vi "I2C_WriteSlaveDeviceAddress_2.vi"(5 "PostAddressDelay(Ticks)":u32, 7 "HalfCycle(Ticks)":u32, 8 "error in":errorcluster, 9 "R/W_Bit":bool, 10 "10-Bit Address":bool, 11 "AddressBits":u8[](array[numeric])=[0, 0] caption="AddressBytes" format="%.0x") -> (0 "error out":errorcluster, 2 "Status":i16)   [LabVIEW 2019]
doc: "Writes the Slave Device Address Byte (w/the R/W Bit set) out the I2C Bus\n\n<b>Inputs:</b>\n---------------------\n<b>AddressBytes</b> the address of the slave device that the master wants to communicate with.\n\n<b>10-Bit Address</b> boolean control for enabling 10-Bit sddressing scheme (True = Use 10-Bit address)\n\n<b>R/W_Bit</b> boolean control for setting the read or write bit (True=Read, =1)\n\n<b>HalfCycle(Ticks)</b> this the number of FPGA clock cycles in half og the clock period. Therefore twice this number yields the clock period, in ticks.\n\n<b>PostAddressDelay(Ticks)</b> the delay in FPGA clock cycles before writing bytes on SDA.\n\n<b>Outputs:</b>\n---------------------\n<b>Status</b> returns a numeric value representing the status of the I2C bus / slave device.\n0 = slave responded\n5002 = slave did not respond\n\nSee block diagram for more details on the implementation details.\n\nAuthor:\nPeter Fuller\nSenior Engineer\nPLF Consulting, LLC\n\nemail: peter@plfconsulting.com\nphone: 617.699.2201"
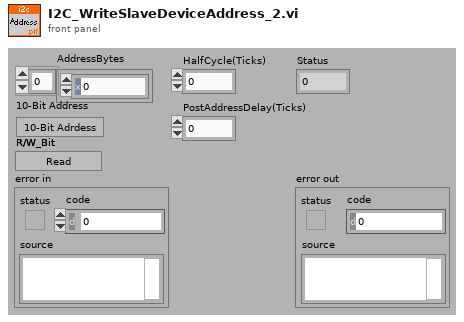
[diagram p1: front panel]
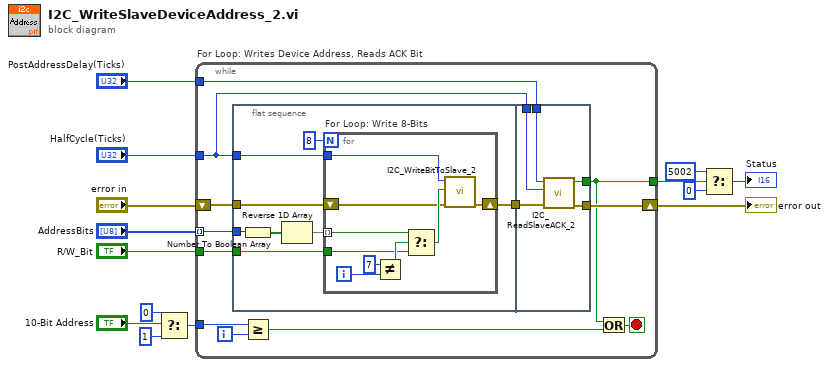
[diagram p0: block diagram]
diagram:
  n1 = Select(t=0, s="10-Bit Address", f=1) -> (s? t:f=w9:i32)
  n2 = while "For Loop: Writes Device Address, Reads ACK Bit" {
    tunnel: "HalfCycle(Ticks)" -> [w18]
    shift-right: [w16] -> w13
    shift-left: "error in" -> [w26]
    tunnel: "AddressBits" -> [w25] mode=indexing
    tunnel: [w15] -> w2
    tunnel: w9 -> [w20]
    tunnel: "R/W_Bit" -> [w19]
    tunnel: "PostAddressDelay(Ticks)" -> [w17]
    i -> [w24]
    stop <- w23 stop-if-true
    n3 = flat-sequence {
      tunnel: w18 -> [w28]
      tunnel: w26 -> [w30]
      tunnel: w25 -> [w33]
      tunnel: [w29] -> w21
      tunnel: w19 -> [w27]
      tunnel: w21 -> [w46]
      tunnel: w18 -> [w48]
      tunnel: w17 -> [w47]
      tunnel: [w45] -> w16
      tunnel: [w44] -> w15
      frame #0 {
        n4 = Number To Boolean Array(number=w33) -> (Boolean array=w32:bool[])
        n5 = Reverse 1D Array(array=w32) -> (reversed array=w31:bool[])
        n6 = for "For Loop: Write 8-Bits" {
          N: 8 -> [_]
          tunnel: w31 -> [w40] mode=indexing
          shift-right: [w35] -> w29
          shift-left: w30 -> [w36]
          tunnel: w28 -> [w43]
          tunnel: w27 -> [w37]
          i -> [w42]
          n7 = Not Equal?(x=7, y=w42) -> (x != y?=w38:bool)
          n8 = Select(t=w40, s=w38, f=w37) -> (s? t:f=w39:bool)
          n9 = call "I2C_WriteBitToSlave_2.vi"("error in"=w36, "Bit_Value"=w39, "HalfCycle(Ticks)"=w43) -> ("error out"=w35:errorcluster)  [unwired: 8 in]
        }
      }
      frame #1 {
        n10 = call "I2C_ReadSlaveACK_2.vi"("error in"=w46, "HalfCycle(Ticks)"=w48, "InterByteTransmitDelay(Ticks)"=w47) -> ("error out"=w45:errorcluster, "SDA"=w44:bool)  [unwired: 7 in]
      }
    }
    n11 = Greater Or Equal?(x=w20, y=w24) -> (x >= y?=w22:bool)
    n12 = Or(x=w15, y=w22) -> (x .or. y?=w23:bool)
  }
  "error out" <- w13
  n13 = Select(t=i16 5002, s=w2, f=i16 0) -> (s? t:f=→"Status":i16)
